vi "main(Test DQMH modules).vi"() -> ()   [LabVIEW 2018, in "Application.lvlib"] (continued)
        n4199 = Bundle By Name(cluster=w9124, "command"="MEAS.mux10-1", "command data"=w9130) -> (w9119:T11)
        n4200 = Bundle By Name(cluster=w9124, "command"="MEAS.mux6_1", "command data"=w9128) -> (w9118:T11)
        n4201 = Bundle By Name(cluster=w9124, "command"="MEAS.demux1-10", "command data"=w9125) -> (w9117:T11)
        n4202 = Bundle By Name(cluster=w9124, "command"="MEAS.eMIC", "command data"=w9121) -> (w9116:T11)
        n4203 = Bundle By Name(cluster=w9124, "command"="MEAS.AllRelaysOFF") -> (w9120:T11)
        n4204 = Build Array(w9120, w9119, w9118, w9117, w9116) -> (w9111:T11[])
        n4205 = Bundle By Name(cluster=w9098, "command"="MEAS.requestAC", "command data"=w9091) -> (w9112:T11)
        n4206 = Bundle By Name(cluster=w9098, "command"="Apps.WaitForEvent", "command data"=w9091) -> (w9097:T11)
        n4207 = Bundle By Name(cluster=w9098, "command"="MEAS.DMM dual read") -> (w9113:T11)
        n4208 = Bundle By Name(cluster=w9098, "command"="Apps.UI Update 1") -> (w9099:T11)
        n4209 = Build Array(w9113, w9112, w9097, w9099) -> (w9110:T11[])
        n4210 = Build Array (concatenate)(w9111, w9110) -> (w9109:T11[])
        n4211 = for {
          tunnel: w9109 -> [w9146] mode=indexing
          tunnel: w9104 -> [w9147]
          tunnel: [w9143] -> w9107 mode=indexing
          n4212 = Unbundle By Name(w9146) -> ("command"=w9145:string, "command data"=w9144:variant)
          n4213 = call "App enquece.vi"("command data"=w9144, "command"=w9145, "queue in"=w9147) -> ("error out"=w9143:errorcluster)  [unwired: 7 in, 1 out]
        }
        n4214 = Merge Errors(w9108, w9107) -> (w9106:errorcluster)
      }
      frame "Test DRV 55A" {
        w9155 = T11 {"command"="", "command data"=variant} ("element")
        w9148 = 55 ("DUT index(0-59)")
        w9181 = T11 {"command"="", "command data"=variant} ("element")
        n4215 = disable-structure shown="LOGGING==TRUE" {
          disable-tunnel: w9159 -> [w9196 _]
          frame condition #0 (active) {
            n4216 = Empty String/Path?(string/path=w9196) -> (empty?=w9199:bool)
            n4217 = Select(t="Quece timeout", s=w9199, f=w9196) -> (s? t:f=w9195:string)
            n4218 = call "string log (SubVI).vi"("Enum"=enum16{"Init", "Log", "Read"}."Log", "state Name"=w9195) -> ()  [unwired: 8 in, 2 out]
          }
          frame condition #1 {
          }
        }
        n4219 = Flush Queue(queue=w9160) -> (queue out=w9161:refnum<queue>)  [unwired: 1 in, 2 out]
        n4220 = Decrement(x=w9148) -> (x-1=w9152:i32)
        n4221 = Index Array(array=w9149, index=w9152) -> (element=w9150:refnum<vi>)
        n4222 = property class="ColBox"(reference=w9150, "Value"=u32 10000536 ("DRV 1")) -> ()  [unwired: 1 in, 2 out]
        n4223 = To Variant(anything=bool[] [TRUE, FALSE, FALSE, FALSE, FALSE, FALSE]) -> (Variant=w9178:variant)
        n4224 = To Variant(anything=T6."demux1_10_channel10" ("demux1_10(x6)_encode")) -> (Variant=w9182:variant)
        n4225 = To Variant(anything=T4."mux6_1_channel1_3" ("mux6_1(3wires)_encode")) -> (Variant=w9185:variant)
        n4226 = To Variant(anything=T5."mux10_1_channel10" ("mux10_1(x6)_encode")) -> (Variant=w9187:variant)
        n4227 = Bundle By Name(cluster=w9181, "command"="MEAS.mux10-1", "command data"=w9187) -> (w9176:T11)
        n4228 = Bundle By Name(cluster=w9181, "command"="MEAS.mux6_1", "command data"=w9185) -> (w9175:T11)
        n4229 = Bundle By Name(cluster=w9181, "command"="MEAS.demux1-10", "command data"=w9182) -> (w9174:T11)
        n4230 = Bundle By Name(cluster=w9181, "command"="MEAS.eMIC", "command data"=w9178) -> (w9173:T11)
        n4231 = Bundle By Name(cluster=w9181, "command"="MEAS.AllRelaysOFF") -> (w9177:T11)
        n4232 = Build Array(w9177, w9176, w9175, w9174, w9173) -> (w9168:T11[])
        n4233 = Bundle By Name(cluster=w9155, "command"="MEAS.requestAC", "command data"=w9148) -> (w9169:T11)
        n4234 = Bundle By Name(cluster=w9155, "command"="Apps.WaitForEvent", "command data"=w9148) -> (w9154:T11)
        n4235 = Bundle By Name(cluster=w9155, "command"="MEAS.DMM dual read") -> (w9170:T11)
        n4236 = Bundle By Name(cluster=w9155, "command"="Apps.UI Update 1") -> (w9156:T11)
        n4237 = Build Array(w9170, w9169, w9154, w9156) -> (w9167:T11[])
        n4238 = Build Array (concatenate)(w9168, w9167) -> (w9166:T11[])
        n4239 = for {
          tunnel: w9166 -> [w9203] mode=indexing
          tunnel: w9161 -> [w9204]
          tunnel: [w9200] -> w9164 mode=indexing
          n4240 = Unbundle By Name(w9203) -> ("command"=w9202:string, "command data"=w9201:variant)
          n4241 = call "App enquece.vi"("command data"=w9201, "command"=w9202, "queue in"=w9204) -> ("error out"=w9200:errorcluster)  [unwired: 7 in, 1 out]
        }
        n4242 = Merge Errors(w9165, w9164) -> (w9163:errorcluster)
      }
      frame "Test DRV 56A" {
        w9212 = T11 {"command"="", "command data"=variant} ("element")
        w9205 = 56 ("DUT index(0-59)")
        w9238 = T11 {"command"="", "command data"=variant} ("element")
        n4243 = disable-structure shown="LOGGING==TRUE" {
          disable-tunnel: w9216 -> [w9253 _]
          frame condition #0 (active) {
            n4244 = Empty String/Path?(string/path=w9253) -> (empty?=w9256:bool)
            n4245 = Select(t="Quece timeout", s=w9256, f=w9253) -> (s? t:f=w9252:string)
            n4246 = call "string log (SubVI).vi"("Enum"=enum16{"Init", "Log", "Read"}."Log", "state Name"=w9252) -> ()  [unwired: 8 in, 2 out]
          }
          frame condition #1 {
          }
        }
        n4247 = Flush Queue(queue=w9217) -> (queue out=w9218:refnum<queue>)  [unwired: 1 in, 2 out]
        n4248 = Decrement(x=w9205) -> (x-1=w9209:i32)
        n4249 = Index Array(array=w9206, index=w9209) -> (element=w9207:refnum<vi>)
        n4250 = property class="ColBox"(reference=w9207, "Value"=u32 10000536 ("DRV 1")) -> ()  [unwired: 1 in, 2 out]
        n4251 = To Variant(anything=bool[] [FALSE, TRUE, FALSE, FALSE, FALSE, FALSE]) -> (Variant=w9235:variant)
        n4252 = To Variant(anything=T6."demux1_10_channel10" ("demux1_10(x6)_encode")) -> (Variant=w9239:variant)
        n4253 = To Variant(anything=T4."mux6_1_channel2_3" ("mux6_1(3wires)_encode")) -> (Variant=w9242:variant)
        n4254 = To Variant(anything=T5."mux10_1_channel10" ("mux10_1(x6)_encode")) -> (Variant=w9244:variant)
        n4255 = Bundle By Name(cluster=w9238, "command"="MEAS.mux10-1", "command data"=w9244) -> (w9233:T11)
        n4256 = Bundle By Name(cluster=w9238, "command"="MEAS.mux6_1", "command data"=w9242) -> (w9232:T11)
        n4257 = Bundle By Name(cluster=w9238, "command"="MEAS.demux1-10", "command data"=w9239) -> (w9231:T11)
        n4258 = Bundle By Name(cluster=w9238, "command"="MEAS.eMIC", "command data"=w9235) -> (w9230:T11)
        n4259 = Bundle By Name(cluster=w9238, "command"="MEAS.AllRelaysOFF") -> (w9234:T11)
        n4260 = Build Array(w9234, w9233, w9232, w9231, w9230) -> (w9225:T11[])
        n4261 = Bundle By Name(cluster=w9212, "command"="MEAS.requestAC", "command data"=w9205) -> (w9226:T11)
        n4262 = Bundle By Name(cluster=w9212, "command"="Apps.WaitForEvent", "command data"=w9205) -> (w9211:T11)
        n4263 = Bundle By Name(cluster=w9212, "command"="MEAS.DMM dual read") -> (w9227:T11)
        n4264 = Bundle By Name(cluster=w9212, "command"="Apps.UI Update 1") -> (w9213:T11)
        n4265 = Build Array(w9227, w9226, w9211, w9213) -> (w9224:T11[])
        n4266 = Build Array (concatenate)(w9225, w9224) -> (w9223:T11[])
        n4267 = for {
          tunnel: w9223 -> [w9260] mode=indexing
          tunnel: w9218 -> [w9261]
          tunnel: [w9257] -> w9221 mode=indexing
          n4268 = Unbundle By Name(w9260) -> ("command"=w9259:string, "command data"=w9258:variant)
          n4269 = call "App enquece.vi"("command data"=w9258, "command"=w9259, "queue in"=w9261) -> ("error out"=w9257:errorcluster)  [unwired: 7 in, 1 out]
        }
        n4270 = Merge Errors(w9222, w9221) -> (w9220:errorcluster)
      }
      frame "Test DRV 57A" {
        w9265 = T11 {"command"="", "command data"=variant} ("element")
        w9266 = 57 ("DUT index(0-59)")
        w9297 = T11 {"command"="", "command data"=variant} ("element")
        n4271 = disable-structure shown="LOGGING==TRUE" {
          disable-tunnel: w9276 -> [w9312 _]
          frame condition #0 (active) {
            n4272 = Empty String/Path?(string/path=w9312) -> (empty?=w9315:bool)
            n4273 = Select(t="Quece timeout", s=w9315, f=w9312) -> (s? t:f=w9311:string)
            n4274 = call "string log (SubVI).vi"("Enum"=enum16{"Init", "Log", "Read"}."Log", "state Name"=w9311) -> ()  [unwired: 8 in, 2 out]
          }
          frame condition #1 {
          }
        }
        n4275 = Flush Queue(queue=w9277) -> (queue out=w9278:refnum<queue>)  [unwired: 1 in, 2 out]
        n4276 = Decrement(x=w9266) -> (x-1=w9270:i32)
        n4277 = Index Array(array=w9267, index=w9270) -> (element=w9268:refnum<vi>)
        n4278 = property class="ColBox"(reference=w9268, "Value"=u32 10000536 ("DRV 1")) -> ()  [unwired: 1 in, 2 out]
        n4279 = To Variant(anything=bool[] [FALSE, FALSE, TRUE, FALSE, FALSE, FALSE]) -> (Variant=w9294:variant)
        n4280 = To Variant(anything=T6."demux1_10_channel10" ("demux1_10(x6)_encode")) -> (Variant=w9298:variant)
        n4281 = To Variant(anything=T4."mux6_1_channel3_3" ("mux6_1(3wires)_encode")) -> (Variant=w9301:variant)
        n4282 = To Variant(anything=T5."mux10_1_channel10" ("mux10_1(x6)_encode")) -> (Variant=w9303:variant)
        n4283 = Bundle By Name(cluster=w9297, "command"="MEAS.mux10-1", "command data"=w9303) -> (w9292:T11)
        n4284 = Bundle By Name(cluster=w9297, "command"="MEAS.mux6_1", "command data"=w9301) -> (w9291:T11)
        n4285 = Bundle By Name(cluster=w9297, "command"="MEAS.demux1-10", "command data"=w9298) -> (w9290:T11)
        n4286 = Bundle By Name(cluster=w9297, "command"="MEAS.eMIC", "command data"=w9294) -> (w9289:T11)
        n4287 = Bundle By Name(cluster=w9297, "command"="MEAS.AllRelaysOFF") -> (w9293:T11)
        n4288 = Build Array(w9293, w9292, w9291, w9290, w9289) -> (w9285:T11[])
        n4289 = Bundle By Name(cluster=w9265, "command"="MEAS.requestAC", "command data"=w9266) -> (w9286:T11)
        n4290 = Bundle By Name(cluster=w9265, "command"="Apps.WaitForEvent", "command data"=w9266) -> (w9272:T11)
        n4291 = Bundle By Name(cluster=w9265, "command"="MEAS.DMM dual read") -> (w9263:T11)
        n4292 = Bundle By Name(cluster=w9265, "command"="WaitFor") -> (w9262:T11)
        n4293 = Bundle By Name(cluster=w9265, "command"="Apps.UI Update 1") -> (w9273:T11)
        n4294 = Build Array(w9263, w9262, w9286, w9272, w9273) -> (w9284:T11[])
        n4295 = Build Array (concatenate)(w9285, w9284) -> (w9283:T11[])
        n4296 = for {
          tunnel: w9283 -> [w9319] mode=indexing
          tunnel: w9278 -> [w9320]
          tunnel: [w9316] -> w9281 mode=indexing
          n4297 = Unbundle By Name(w9319) -> ("command"=w9318:string, "command data"=w9317:variant)
          n4298 = call "App enquece.vi"("command data"=w9317, "command"=w9318, "queue in"=w9320) -> ("error out"=w9316:errorcluster)  [unwired: 7 in, 1 out]
        }
        n4299 = Merge Errors(w9282, w9281) -> (w9280:errorcluster)
      }
      frame "Test DRV 58A" {
        w9324 = T11 {"command"="", "command data"=variant} ("element")
        w9325 = 58 ("DUT index(0-59)")
        w9356 = T11 {"command"="", "command data"=variant} ("element")
        n4300 = disable-structure shown="LOGGING==TRUE" {
          disable-tunnel: w9335 -> [w9371 _]
          frame condition #0 (active) {
            n4301 = Empty String/Path?(string/path=w9371) -> (empty?=w9374:bool)
            n4302 = Select(t="Quece timeout", s=w9374, f=w9371) -> (s? t:f=w9370:string)
            n4303 = call "string log (SubVI).vi"("Enum"=enum16{"Init", "Log", "Read"}."Log", "state Name"=w9370) -> ()  [unwired: 8 in, 2 out]
          }
          frame condition #1 {
          }
        }
        n4304 = Flush Queue(queue=w9336) -> (queue out=w9337:refnum<queue>)  [unwired: 1 in, 2 out]
        n4305 = Decrement(x=w9325) -> (x-1=w9329:i32)
        n4306 = Index Array(array=w9326, index=w9329) -> (element=w9327:refnum<vi>)
        n4307 = property class="ColBox"(reference=w9327, "Value"=u32 10000536 ("DRV 1")) -> ()  [unwired: 1 in, 2 out]
        n4308 = To Variant(anything=bool[] [FALSE, FALSE, FALSE, TRUE, FALSE, FALSE]) -> (Variant=w9353:variant)
        n4309 = To Variant(anything=T6."demux1_10_channel10" ("demux1_10(x6)_encode")) -> (Variant=w9357:variant)
        n4310 = To Variant(anything=T4."mux6_1_channel4_3" ("mux6_1(3wires)_encode")) -> (Variant=w9360:variant)
        n4311 = To Variant(anything=T5."mux10_1_channel10" ("mux10_1(x6)_encode")) -> (Variant=w9362:variant)
        n4312 = Bundle By Name(cluster=w9356, "command"="MEAS.mux10-1", "command data"=w9362) -> (w9351:T11)
        n4313 = Bundle By Name(cluster=w9356, "command"="MEAS.mux6_1", "command data"=w9360) -> (w9350:T11)
        n4314 = Bundle By Name(cluster=w9356, "command"="MEAS.demux1-10", "command data"=w9357) -> (w9349:T11)
        n4315 = Bundle By Name(cluster=w9356, "command"="MEAS.eMIC", "command data"=w9353) -> (w9348:T11)
        n4316 = Bundle By Name(cluster=w9356, "command"="MEAS.AllRelaysOFF") -> (w9352:T11)
        n4317 = Build Array(w9352, w9351, w9350, w9349, w9348) -> (w9344:T11[])
        n4318 = Bundle By Name(cluster=w9324, "command"="MEAS.requestAC", "command data"=w9325) -> (w9345:T11)
        n4319 = Bundle By Name(cluster=w9324, "command"="Apps.WaitForEvent", "command data"=w9325) -> (w9331:T11)
        n4320 = Bundle By Name(cluster=w9324, "command"="MEAS.DMM dual read") -> (w9323:T11)
        n4321 = Bundle By Name(cluster=w9324, "command"="WaitFor") -> (w9322:T11)
        n4322 = Bundle By Name(cluster=w9324, "command"="Apps.UI Update 1") -> (w9332:T11)
        n4323 = Build Array(w9323, w9322, w9345, w9331, w9332) -> (w9343:T11[])
        n4324 = Build Array (concatenate)(w9344, w9343) -> (w9342:T11[])
        n4325 = for {
          tunnel: w9342 -> [w9378] mode=indexing
          tunnel: w9337 -> [w9379]
          tunnel: [w9375] -> w9340 mode=indexing
          n4326 = Unbundle By Name(w9378) -> ("command"=w9377:string, "command data"=w9376:variant)
          n4327 = call "App enquece.vi"("command data"=w9376, "command"=w9377, "queue in"=w9379) -> ("error out"=w9375:errorcluster)  [unwired: 7 in, 1 out]
        }
        n4328 = Merge Errors(w9341, w9340) -> (w9339:errorcluster)
      }
      frame "Test DRV 59A" {
        w9383 = T11 {"command"="", "command data"=variant} ("element")
        w9384 = 59 ("DUT index(0-59)")
        w9415 = T11 {"command"="", "command data"=variant} ("element")
        n4329 = disable-structure shown="LOGGING==TRUE" {
          disable-tunnel: w9394 -> [w9430 _]
          frame condition #0 (active) {
            n4330 = Empty String/Path?(string/path=w9430) -> (empty?=w9433:bool)
            n4331 = Select(t="Quece timeout", s=w9433, f=w9430) -> (s? t:f=w9429:string)
            n4332 = call "string log (SubVI).vi"("Enum"=enum16{"Init", "Log", "Read"}."Log", "state Name"=w9429) -> ()  [unwired: 8 in, 2 out]
          }
          frame condition #1 {
          }
        }
        n4333 = Flush Queue(queue=w9395) -> (queue out=w9396:refnum<queue>)  [unwired: 1 in, 2 out]
        n4334 = Decrement(x=w9384) -> (x-1=w9388:i32)
        n4335 = Index Array(array=w9385, index=w9388) -> (element=w9386:refnum<vi>)
        n4336 = property class="ColBox"(reference=w9386, "Value"=u32 10000536 ("DRV 1")) -> ()  [unwired: 1 in, 2 out]
        n4337 = To Variant(anything=T5."mux10_1_channel10" ("mux10_1(x6)_encode")) -> (Variant=w9421:variant)
        n4338 = To Variant(anything=T4."mux6_1_channel5_3" ("mux6_1(3wires)_encode")) -> (Variant=w9419:variant)
        n4339 = To Variant(anything=T6."demux1_10_channel10" ("demux1_10(x6)_encode")) -> (Variant=w9416:variant)
        n4340 = To Variant(anything=bool[] [FALSE, FALSE, FALSE, FALSE, TRUE, FALSE]) -> (Variant=w9412:variant)
        n4341 = Bundle By Name(cluster=w9415, "command"="MEAS.mux10-1", "command data"=w9421) -> (w9410:T11)
        n4342 = Bundle By Name(cluster=w9415, "command"="MEAS.mux6_1", "command data"=w9419) -> (w9409:T11)
        n4343 = Bundle By Name(cluster=w9415, "command"="MEAS.demux1-10", "command data"=w9416) -> (w9408:T11)
        n4344 = Bundle By Name(cluster=w9415, "command"="MEAS.eMIC", "command data"=w9412) -> (w9407:T11)
        n4345 = Bundle By Name(cluster=w9415, "command"="MEAS.AllRelaysOFF") -> (w9411:T11)
        n4346 = Build Array(w9411, w9410, w9409, w9408, w9407) -> (w9403:T11[])
        n4347 = Bundle By Name(cluster=w9383, "command"="MEAS.requestAC", "command data"=w9384) -> (w9404:T11)
        n4348 = Bundle By Name(cluster=w9383, "command"="Apps.WaitForEvent", "command data"=w9384) -> (w9390:T11)
        n4349 = Bundle By Name(cluster=w9383, "command"="MEAS.DMM dual read") -> (w9382:T11)
        n4350 = Bundle By Name(cluster=w9383, "command"="WaitFor") -> (w9381:T11)
        n4351 = Bundle By Name(cluster=w9383, "command"="Apps.UI Update 1") -> (w9391:T11)
        n4352 = Build Array(w9382, w9381, w9404, w9390, w9391) -> (w9402:T11[])
        n4353 = Build Array (concatenate)(w9403, w9402) -> (w9401:T11[])
        n4354 = for {
          tunnel: w9401 -> [w9437] mode=indexing
          tunnel: w9396 -> [w9438]
          tunnel: [w9434] -> w9399 mode=indexing
          n4355 = Unbundle By Name(w9437) -> ("command"=w9436:string, "command data"=w9435:variant)
          n4356 = call "App enquece.vi"("command data"=w9435, "command"=w9436, "queue in"=w9438) -> ("error out"=w9434:errorcluster)  [unwired: 7 in, 1 out]
        }
        n4357 = Merge Errors(w9400, w9399) -> (w9398:errorcluster)
      }
      frame "Test DRV 60A" {
        w9440 = T11 {"command"="", "command data"=variant} ("element")
        w9443 = 60 ("DUT index(0-59)")
        w9474 = T11 {"command"="", "command data"=variant} ("element")
        n4358 = disable-structure shown="LOGGING==TRUE" {
          disable-tunnel: w9453 -> [w9489 _]
          frame condition #0 (active) {
            n4359 = Empty String/Path?(string/path=w9489) -> (empty?=w9492:bool)
            n4360 = Select(t="Quece timeout", s=w9492, f=w9489) -> (s? t:f=w9488:string)
            n4361 = call "string log (SubVI).vi"("Enum"=enum16{"Init", "Log", "Read"}."Log", "state Name"=w9488) -> ()  [unwired: 8 in, 2 out]
          }
          frame condition #1 {
          }
        }
        n4362 = Flush Queue(queue=w9454) -> (queue out=w9455:refnum<queue>)  [unwired: 1 in, 2 out]
        n4363 = Decrement(x=w9443) -> (x-1=w9447:i32)
        n4364 = Index Array(array=w9444, index=w9447) -> (element=w9445:refnum<vi>)
        n4365 = property class="ColBox"(reference=w9445, "Value"=u32 10000536 ("DRV 1")) -> ()  [unwired: 1 in, 2 out]
        n4366 = To Variant(anything=bool[] [FALSE, FALSE, FALSE, FALSE, FALSE, TRUE]) -> (Variant=w9471:variant)
        n4367 = To Variant(anything=T6."demux1_10_channel10" ("demux1_10(x6)_encode")) -> (Variant=w9475:variant)
        n4368 = To Variant(anything=T4."mux6_1_channel6_3" ("mux6_1(3wires)_encode")) -> (Variant=w9478:variant)
        n4369 = To Variant(anything=T5."mux10_1_channel10" ("mux10_1(x6)_encode")) -> (Variant=w9480:variant)
        n4370 = Bundle By Name(cluster=w9474, "command"="MEAS.mux10-1", "command data"=w9480) -> (w9469:T11)
        n4371 = Bundle By Name(cluster=w9474, "command"="MEAS.mux6_1", "command data"=w9478) -> (w9468:T11)
        n4372 = Bundle By Name(cluster=w9474, "command"="MEAS.demux1-10", "command data"=w9475) -> (w9467:T11)
        n4373 = Bundle By Name(cluster=w9474, "command"="MEAS.eMIC", "command data"=w9471) -> (w9466:T11)
        n4374 = Bundle By Name(cluster=w9474, "command"="MEAS.AllRelaysOFF") -> (w9470:T11)
        n4375 = Build Array(w9470, w9469, w9468, w9467, w9466) -> (w9462:T11[])
        n4376 = Bundle By Name(cluster=w9440, "command"="MEAS.requestAC", "command data"=w9443) -> (w9463:T11)
        n4377 = Bundle By Name(cluster=w9440, "command"="Apps.WaitForEvent", "command data"=w9443) -> (w9449:T11)
        n4378 = Bundle By Name(cluster=w9440, "command"="MEAS.DMM dual read") -> (w9441:T11)
        n4379 = Bundle By Name(cluster=w9440, "command"="WaitFor") -> (w9439:T11)
        n4380 = Bundle By Name(cluster=w9440, "command"="Apps.UI Update 1") -> (w9450:T11)
        n4381 = Build Array(w9441, w9439, w9463, w9449, w9450) -> (w9461:T11[])
        n4382 = Build Array (concatenate)(w9462, w9461) -> (w9460:T11[])
        n4383 = for {
          tunnel: w9460 -> [w9496] mode=indexing
          tunnel: w9455 -> [w9497]
          tunnel: [w9493] -> w9458 mode=indexing
          n4384 = Unbundle By Name(w9496) -> ("command"=w9495:string, "command data"=w9494:variant)
          n4385 = call "App enquece.vi"("command data"=w9494, "command"=w9495, "queue in"=w9497) -> ("error out"=w9493:errorcluster)  [unwired: 7 in, 1 out]
        }
        n4386 = Merge Errors(w9459, w9458) -> (w9457:errorcluster)
      }
    }
    "DC Measure Completed" <- w230
    "Progress" <- w227
    n4387 = feedback-in #1(w227) -> ()
    n4388 = disable-structure shown="LOGGING==TRUE" {
      disable-tunnel: [w254 _] -> w228
      disable-tunnel: w229 -> [w251 _]
      frame condition #0 (active) {
        n4389 = property on="State log" class="Str"("Text.Scroll Position"=inf) -> ()  [unwired: 2 in, 2 out]
        n4390 = call "string log (SubVI).vi"("error in (no error)"=w251, "Enum"=enum16{"Init", "Log", "Read"}."Read") -> ("error out"=w254:errorcluster, "State log"=→"State log":string)  [unwired: 8 in]
      }
      frame condition #1 {
      }
    }
  }
  n4391 = disable-structure shown="Disabled" {
    frame Disabled {
      n4392 = case shown="\"00037845(M26)\"" "Enum" {
        tunnel: [w9507 w9524 w9535 w9554] -> _
        frame "All DRV" {
          n4393 = Build Array("Test Shorted Circuits", "Timer Start", "Test Channel 1", "Test Channel 2", "Test Channel 3", "Test Channel 4", "Test Channel 5", "Test Channel 6") -> (w9499:string[])
          n4394 = Build Array("Test Channel 7", "Test Channel 8", "Test Channel 9", "Test Channel 10", "Timer Stop") -> (w9508:string[])
          n4395 = Build Array("MEAS.AllRelaysOFF", "MEAS.Reset JIG", "Apps.UI Update 2") -> (w9500:string[])
          n4396 = Build Array (concatenate)(w9499, w9508, w9500) -> (w9507:string[])
        }
        frame "Fixxed" {
          n4397 = Build Array("Test Shorted Circuits", "Timer Start", "Test Channel 1", "Test Channel 2", "Test Channel 3", "Test Channel 4", "Test Channel 5", "Test Channel 6", "Test Channel 7") -> (w9526:string[])
          n4398 = Build Array("MEAS.AllRelaysOFF", "MEAS.Reset JIG", "Apps.UI Update 2") -> (w9520:string[])
          n4399 = Build Array (concatenate)(w9526, "Timer Stop", w9520) -> (w9524:string[])
        }
        frame "Pinpoint_JIG" {
          n4400 = Build Array("Test Channel 8", "Test Channel 9", "Test Channel 10") -> (w9539:string[])
          n4401 = Build Array("Test Shorted Circuits", "Timer Start") -> (w9536:string[])
          n4402 = Build Array("MEAS.AllRelaysOFF", "MEAS.Reset JIG", "Apps.UI Update 2") -> (w9538:string[])
          n4403 = Build Array (concatenate)(w9536, w9539, "Timer Stop", w9538) -> (w9535:string[])
        }
        frame "00037845(M26)" {
          n4404 = Build Array("Test Shorted Circuits", "Timer Start") -> (w9555:string[])
          n4405 = Build Array("Test Channel 8", "Test Channel 9", "Test Channel 10A", "Timer Stop") -> (w9549:string[])
          n4406 = Build Array("MEAS.AllRelaysOFF", "MEAS.Reset JIG", "Apps.UI Update 2") -> (w9548:string[])
          n4407 = Build Array (concatenate)(w9555, w9549, w9548) -> (w9554:string[])
        }
      }
    }
    frame Enabled {
    }
  }
  n4408 = Unregister For Events(event registration refnum=w94) -> (error out=w10:errorcluster)  [unwired: 1 in]
  n4409 = Release Queue(queue=w90, error in (no error)=w89) -> (error out=w8:errorcluster)  [unwired: 1 in, 2 out]
  n4410 = Destroy User Event(user event=w7, error in=w8) -> (error out=w4:errorcluster)
  n4411 = while {
    shift-right: [w9565] -> w3
    shift-left: w5 -> [w9567]
    shift-right: [w9562] -> w2
    shift-left: w4 -> [w9566]
    stop <- w9563 stop-if-true
    n4412 = Get Queue Status(queue=w9567, error in (no error)=w9566) -> (queue out=w9565:refnum<queue>, error out=w9562:errorcluster, # elements in queue=w9564:i32)  [unwired: 1 in, 5 out]
    n4413 = Equal To 0?(x=w9564) -> (x = 0?=w9563:bool)
    n4414 = Wait (ms)(milliseconds to wait=u32 10) -> ()  [unwired: 1 out]
  }
  n4415 = Release Queue(queue=w3, error in (no error)=w2) -> (error out=w1:errorcluster)  [unwired: 1 in, 2 out]
  n4416 = Merge Errors(w10, w1) -> (w9:errorcluster)
  n4417 = disable-structure shown="RUN_TIME_ENGINE==True" {
    disable-tunnel: w9 -> [w9568 _]
    frame condition #0 (active) {
      "error out" <- w9568
    }
    frame condition #1 {
      n4418 = Quit LabVIEW(quit? (T)=TRUE) -> ()
    }
  }
